vi "Add.vi"(7 "Export VI?":bool, 8 "error in (no error)":errorcluster, 10 "ProjectItem Refnum":refnum<vi>, 11 "DLL in":refnum<class "NI_AB_API_DLL.lvclass">) -> (0 "error out":errorcluster, 3 "DLL out":refnum<class "NI_AB_API_DLL.lvclass">)   [LabVIEW 2020, in "NI_AB_API_DLL.lvclass"]
uses:
  <vilib>/AppBuilder/AB_API/DLL/NI_AB_API_DLL.lvclass
  e:/builds/penguin/labview/branches/2020/dev/dist/vi.lib/AppBuilder/AB_API/Build/NI_AB_API_Build.lvclass
  <vilib>/AppBuilder/AB_Classes/DLL/AB_DLL.lvclass
  e:/builds/penguin/labview/branches/2020/dev/dist/vi.lib/AppBuilder/AB_Classes/Build/AB_Build.lvclass
  <vilib>/AppBuilder/AB_Classes/Source/VI/AB_Source_VI.lvclass
  e:/builds/penguin/labview/branches/2020/dev/dist/vi.lib/AppBuilder/AB_Classes/Source/AB_Source.lvclass
  <vilib>/AppBuilder/AB_Classes/Build/AB_Build.lvclass
  <vilib>/AppBuilder/AB_Classes/Source/AB_Source.lvclass
  <vilib>/AppBuilder/AB_API/Build/NI_AB_API_Build.lvclass
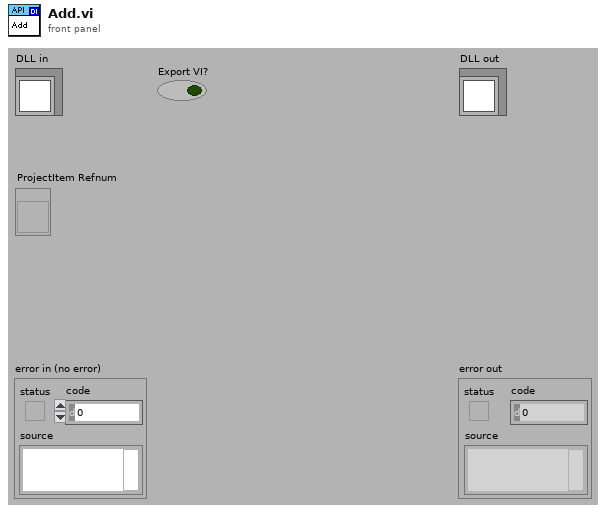
[diagram p1: front panel]
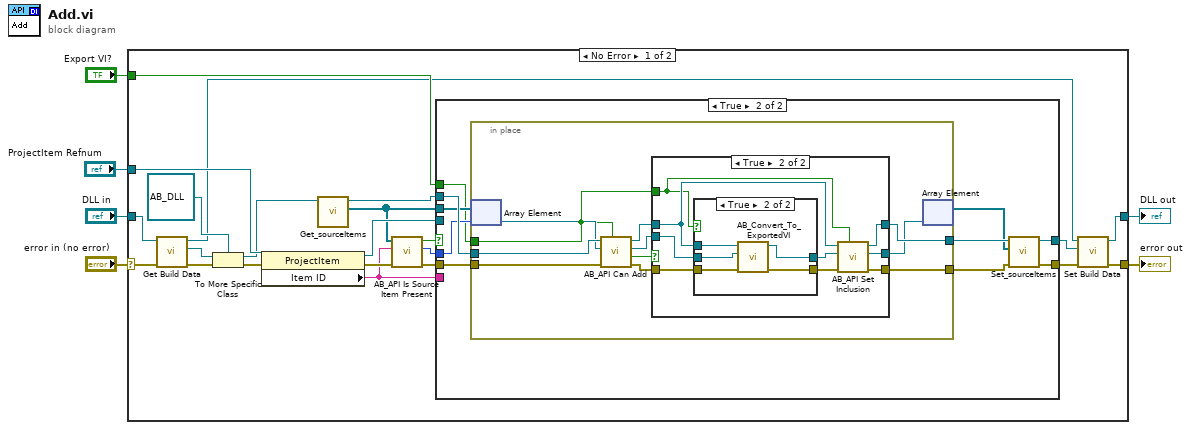
[diagram p0: block diagram]
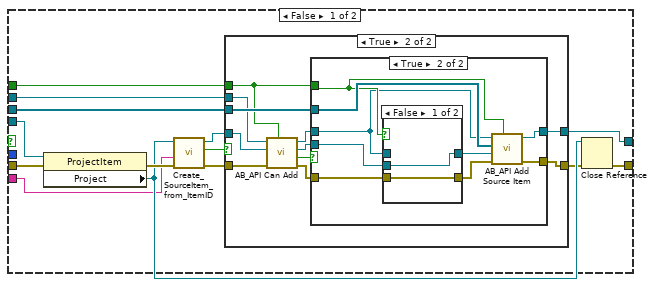
[diagram p2: hidden frame]
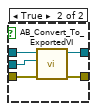
[diagram p5: hidden frame]
diagram:
  n1 = case shown="No Error" "error in (no error)" {
    selector: "error in (no error)" -> [w10 w115]
    tunnel: [w8 w115] -> w5
    tunnel: [w17 w114] -> w3
    tunnel: "DLL in" -> [w15 w114]
    tunnel: "ProjectItem Refnum" -> [w28 _]
    tunnel: "Export VI?" -> [w27 _]
    frame No Error {
      n2 = call <vilib>:"Get Build Data.vi"("error in (no error)"=w10, "NI_AB_API_Build in"=w15) -> ("error out"=w11:errorcluster, "AB_Build.lvclass"=w14:refnum<class "AB_Build.lvclass">, "NI_AB_API_Build out"=w12:refnum<class "NI_AB_API_DLL.lvclass">)  [unwired: 7 in]
      n3 = To More Specific Class(target class=refnum<class "AB_DLL.lvclass"> refnum ("AB_DLL.lvclass"), reference=w14, error in=w11) -> (specific class reference=w13:refnum<class "AB_DLL.lvclass">, error out=w9:errorcluster)
      n4 = property class="ProjectItem"(reference=w28, error in=w9) -> (reference out=w26:refnum<vi>, error out=w21:errorcluster, "Item ID"=w20:string)
      n5 = call <vilib>:"Get_sourceItems.vi"("Class in"=w13) -> ("sourceItems"=w25:refnum<class "AB_Source.lvclass">[], "Class out"=w24:refnum<class "AB_DLL.lvclass">)  [unwired: 8 in, 1 out]
      n6 = call <vilib>:"AB_API Is Source Item Present.vi"("error in"=w21, "item ID"=w20, "source items"=w25) -> ("error out"=w22:errorcluster, "index"=w19:i32, "source item present?"=w23:bool)  [unwired: 6 in]
      n7 = case shown="True" w23 {
        tunnel: w26 -> [w42 _]
        tunnel: [w38 w78] -> w16
        tunnel: [w34 w75] -> w7
        tunnel: w22 -> [w33 w80]
        tunnel: w24 -> [w32 w83]
        tunnel: w20 -> [w31 _]
        tunnel: w25 -> [w30 w82]
        tunnel: w19 -> [_ w81]
        tunnel: w27 -> [w29 w74]
        frame False {
          n8 = property class="ProjectItem"(reference=w42, error in=w33) -> (error out=w41:errorcluster, "Project"=w36:refnum<vi>)  [unwired: 1 out]
          n9 = call <vilib>:"Create_SourceItem_from_ItemID.vi"("error in (no error)"=w41, "itemID"=w31, "Project Refnum"=w36) -> ("error out"=w39:errorcluster, "valid?"=w37:bool, "AB_Source out"=w40:refnum<class "AB_Source.lvclass">)  [unwired: 6 in]
          n10 = case shown="True" w37 {
            tunnel: w40 -> [_ w51]
            tunnel: w39 -> [w43 w50]
            tunnel: w32 -> [w44 w52]
            tunnel: [w44 w55] -> w38
            tunnel: [w43 w54] -> w35
            tunnel: w30 -> [_ w53]
            tunnel: w29 -> [_ w45]
            frame False {
            }
            frame True {
              n11 = call <vilib>:"AB_API Can Add.vi"("top tree? (true)"=w45, "error in (no error)"=w50, "AB_Source in"=w51, "Build in"=w52) -> ("error out"=w46:errorcluster, "can add?"=w49:bool, "AB_Source out"=w47:refnum<class "AB_Source.lvclass">, "Build out"=w48:refnum<class "AB_DLL.lvclass">)  [unwired: 4 in]
              n12 = case shown="True" w49 {
                tunnel: [w56 w64] -> w55
                tunnel: [w57 w65] -> w54
                tunnel: w53 -> [_ w66]
                tunnel: w45 -> [_ w61]
                tunnel: w48 -> [w56 w58]
                tunnel: w47 -> [_ w60]
                tunnel: w46 -> [w57 w59]
                frame False {
                }
                frame True {
                  n13 = case shown="False" w61 {
                    tunnel: [w67 w73] -> w63
                    tunnel: [w68 w72] -> w62
                    tunnel: w58 -> [_ w69]
                    tunnel: w60 -> [w67 w71]
                    tunnel: w59 -> [w68 w70]
                    frame False {
                    }
                    frame True {
                      n14 = call <vilib>:"AB_Convert_To_ExportedVI.vi"("error in (no error)"=w70, "Source in"=w71, "Build in"=w69) -> ("error out"=w72:errorcluster, "Exported VI out"=w73:refnum<class "AB_Source_VI.lvclass">)  [unwired: 7 out]
                    }
                  }
                  n15 = call <vilib>:"AB_API Add Source Item.vi"("top tree? (true)"=w61, "error in"=w62, "Source in"=w63, "source items"=w66, "Build in"=w58) -> ("error out"=w65:errorcluster, "Build out"=w64:refnum<class "AB_DLL.lvclass">)  [unwired: 5 in]
                }
              }
            }
          }
          n16 = Close Reference(reference=w36, error in (no error)=w35) -> (error out=w34:errorcluster)
        }
        frame True {
          n17 = in-place {
            in-place-border: [w94] -> w79
            in-place-border: w83 -> [w91]
            in-place-border: w80 -> [w87]
            in-place-border: [w93] -> w76
            in-place-border: w74 -> [w84]
            n18 = in-place-array #1(w82, w81) -> (w89:refnum<class "AB_Source.lvclass">)
            n19 = call <vilib>:"AB_API Can Add.vi"("top tree? (true)"=w84, "error in (no error)"=w87, "AB_Source in"=w89, "Build in"=w91) -> ("error out"=w86:errorcluster, "can add?"=w85:bool, "AB_Source out"=w88:refnum<class "AB_Source.lvclass">, "Build out"=w90:refnum<class "AB_DLL.lvclass">)  [unwired: 4 in]
            n20 = case shown="True" w85 {
              tunnel: [w95 w104] -> w93
              tunnel: [w97 w106] -> w94
              tunnel: w90 -> [w97 w103]
              tunnel: w88 -> [w96 w102]
              tunnel: w86 -> [w95 w101]
              tunnel: [w96 w105] -> w92
              tunnel: w84 -> [_ w98]
              frame False {
              }
              frame True {
                n21 = case shown="True" w98 {
                  tunnel: w103 -> [_ w113]
                  tunnel: w102 -> [w108 w112]
                  tunnel: [w108 w111] -> w100
                  tunnel: w101 -> [w107 w110]
                  tunnel: [w107 w109] -> w99
                  frame False {
                  }
                  frame True {
                    n22 = call <vilib>:"AB_Convert_To_ExportedVI.vi"("error in (no error)"=w110, "Source in"=w112, "Build in"=w113) -> ("error out"=w109:errorcluster, "Exported VI out"=w111:refnum<class "AB_Source_VI.lvclass">)  [unwired: 7 out]
                  }
                }
                n23 = call <vilib>:"AB_API Set Inclusion.vi"("top tree? (true)"=w98, "error in (no error)"=w99, "Source in"=w100, "Build in"=w103) -> ("error out"=w104:errorcluster, "AB_Source_VI out"=w105:refnum<class "AB_Source.lvclass">, "AB_Build out"=w106:refnum<class "AB_DLL.lvclass">)  [unwired: 5 in]
              }
            }
            n24 = in-place-array #1(w92) -> (w77:refnum<class "AB_Source.lvclass">[])  [unwired: 1 out]
          }
          n25 = call <vilib>:"Set_sourceItems.vi"("error in (no error)"=w76, "sourceItems"=w77, "Class in"=w79) -> ("error out"=w75:errorcluster, "Class out"=w78:refnum<class "AB_DLL.lvclass">)  [unwired: 7 out]
        }
      }
      n26 = call <vilib>:"Set Build Data.vi"("error in (no error)"=w7, "AB_Build.lvclass"=w16, "NI_AB_API_Build in"=w12) -> ("error out"=w8:errorcluster, "NI_AB_API_Build out"=w17:refnum<class "NI_AB_API_DLL.lvclass">)  [unwired: 7 in]
    }
    frame Error {
    }
  }
  "error out" <- w5
  "DLL out" <- w3
